vi "DPO_7k_Default_Setup.vi"(8 "Error in":errorcluster, 11 "VISA resource name in":refnum<visa-resource-name>) -> (0 "Error out":errorcluster, 3 "VISA resource name out":refnum<visa-resource-name>)   [LabVIEW 2020]
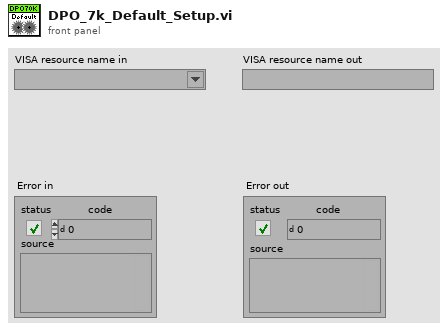
[diagram p1: front panel]
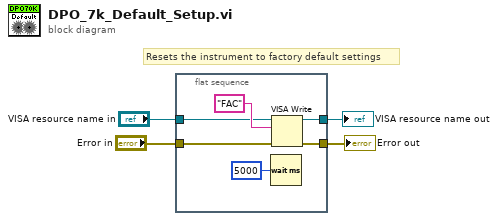
[diagram p0: block diagram]
diagram:
  # "Resets the instrument to factory default settings"
  n1 = flat-sequence {
    tunnel: "VISA resource name in" -> [w8]
    tunnel: "Error in" -> [w7]
    tunnel: [w6] -> w1
    tunnel: [w5] -> w2
    frame #0 {
      n2 = Wait (ms)(milliseconds to wait=u32 5000) -> ()  [unwired: 1 out]
      n3 = VISA Write(VISA resource name=w8, write buffer="FAC", error in (no error)=w7) -> (VISA resource name out=w5:refnum<visa-resource-name>, error out=w6:errorcluster)  [unwired: 1 out]
    }
  }
  "VISA resource name out" <- w2
  "Error out" <- w1
